vi "Digital Input Signals.vi"(8 "error in (no error)":errorcluster, 10 "Digital Input Signals":digitalwaveform[](array[waveform]), 11 "TCP 380 in":refnum<class "TCP 380.lvclass">) -> (0 "error out":errorcluster, 3 "TCP 380 out":refnum<class "TCP 380.lvclass">)   [LabVIEW 2021, in "TCP 380.lvclass"]
uses:
  TCP 380.lvclass
  TCP 380.lvclass/TCP 380.ctl
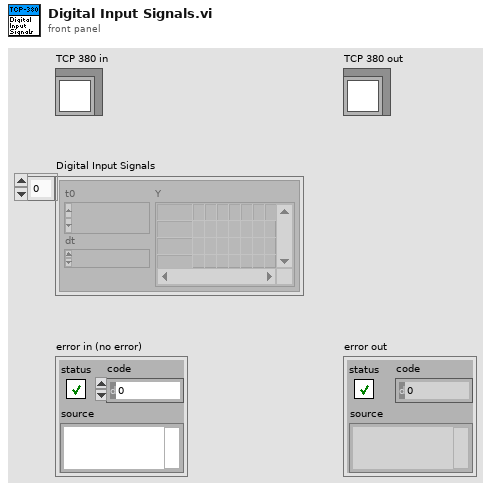
[diagram p1: front panel]
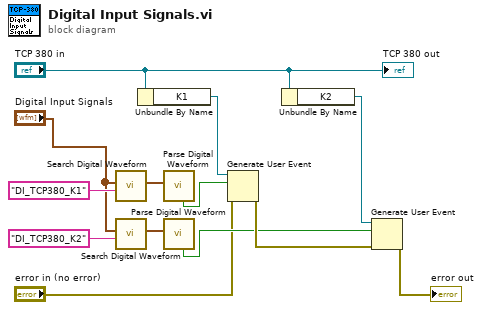
[diagram p0: block diagram]
diagram:
  n1 = call <vilib>:"Search Digital Waveform.vi"("NI_ChannelName"="DI_TCP380_K1" ("key"), "Waveforms"="Digital Input Signals") -> ("Waveform"=w9:digitalwaveform)  [unwired: 8 in, 1 out]
  n2 = call <vilib>:"Search Digital Waveform.vi"("NI_ChannelName"="DI_TCP380_K2" ("key"), "Waveforms"="Digital Input Signals") -> ("Waveform"=w7:digitalwaveform)  [unwired: 8 in, 1 out]
  n3 = Unbundle By Name("TCP 380 in") -> ("K1"=w13:refnum<user-event>)
  n4 = call <vilib>:"Parse Digital Waveform.vi"("Digital Wave"=w9) -> ("Boolean"=w8:bool)  [unwired: 6 in, 4 out]
  n5 = call <vilib>:"Parse Digital Waveform.vi"("Digital Wave"=w7) -> ("Boolean"=w6:bool)  [unwired: 6 in, 4 out]
  n6 = Generate User Event(user event=w13, event data cluster=w8, error in="error in (no error)") -> (error out=w11:errorcluster)  [unwired: 1 in, 1 out]
  n7 = Unbundle By Name("TCP 380 in") -> ("K2"=w12:refnum<user-event>)
  n8 = Generate User Event(user event=w12, event data cluster=w6, error in=w11) -> (error out=→"error out":errorcluster)  [unwired: 1 in, 1 out]
  "TCP 380 out" <- "TCP 380 in"
